vi "configure.vi"(8 "error in (no error)":errorcluster, 11 "DAQmxDigitalOut in":refnum<class "DigitalOutDL110325DAQmx.lvclass">) -> (0 "error out":errorcluster, 3 "DAQmxDigitalOut out":refnum<class "DigitalOutDL110325DAQmx.lvclass">)   [LabVIEW 2010, in "DigitalOutDL110325DAQmx.lvclass"]
doc: "The dynamic dispatch version of this VI loads and displays the configuration file associated with the plug-in object. The user modify and save the configuration data."
uses:
  DigitalOutDL110325DAQmx.lvclass
  DigitalOutDL110325DAQmx.lvclass/DigitalOutDL110325DAQmx.ctl
  common/classes/GenericComponent/GenericComponent/GenericComponent.lvclass
panel:
  out "Configuration":string
  in  "digital output line":tag
  in  "Save Button":bool
  in  "Cancel Button":bool
  # "Configure DAQmxDigitalOut component"
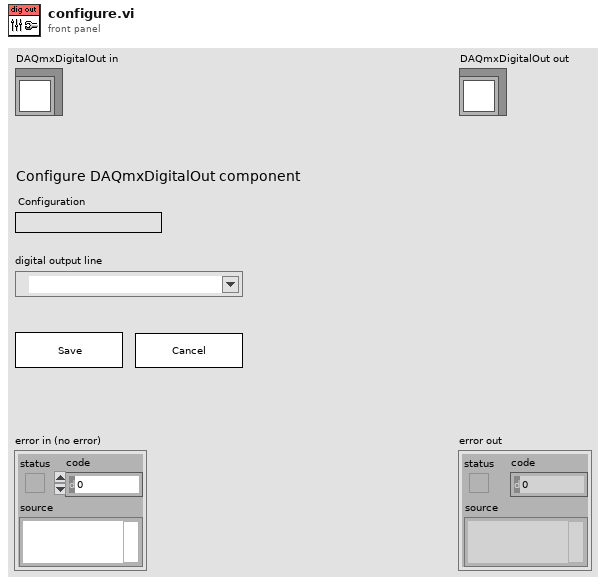
[diagram p1: front panel]
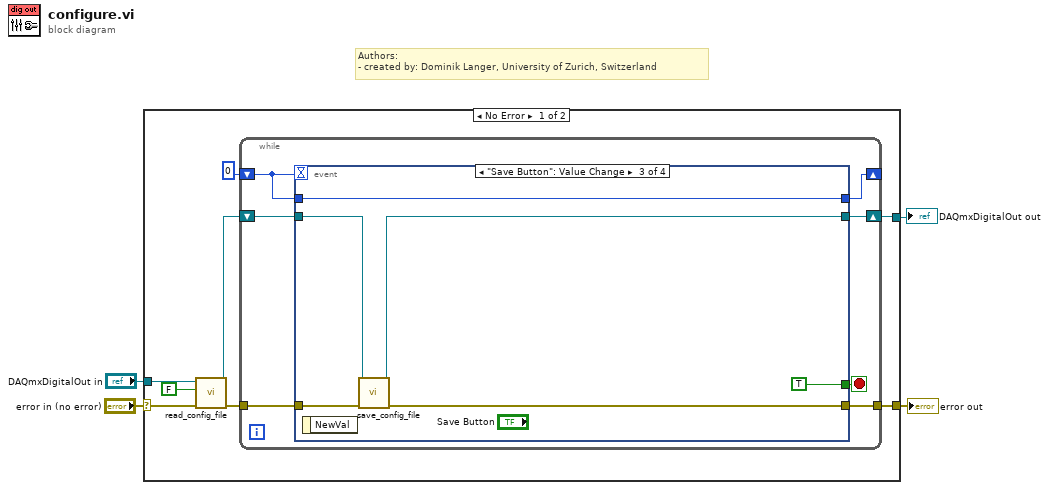
[diagram p0: block diagram]
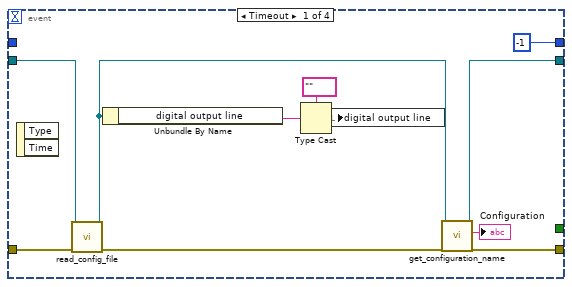
[diagram p2: hidden frame]
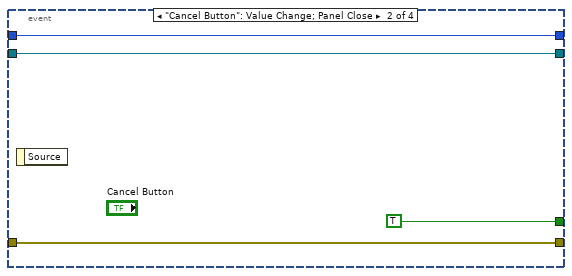
[diagram p3: hidden frame]
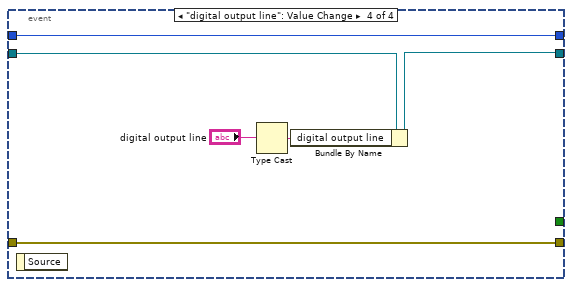
[diagram p4: hidden frame]
diagram:
  # "Authors: \n- created by: Dominik Langer, University of Zurich, Switzerland"
  n1 = case shown="No Error" "error in (no error)" {
    selector: "error in (no error)" -> [w9 w48]
    tunnel: [w12 w48] -> w1
    tunnel: [w10 w47] -> w3
    tunnel: "DAQmxDigitalOut in" -> [w7 w47]
    frame No Error {
      n2 = call-dynamic "read_config_file.vi"("error in (no error)"=w9, "force load?"=FALSE, "GenericPlugin in"=w7) -> ("error out"=w8:errorcluster, "GenericPlugin out"=w6:refnum<class "DigitalOutDL110325DAQmx.lvclass">)  [unwired: 7 out]
      n3 = while {
        tunnel: w8 -> [w19]
        tunnel: [w18] -> w12
        shift-right: [w15] -> _
        shift-left: 0 -> [w16]
        shift-right: [w13] -> w10
        shift-left: w6 -> [w14]
        stop <- w17 stop-if-true
        n4 = event shown="[2] \"Save Button\": Value Change" {
          selector: _ -> [_ _ _ _]
          dyn-events: _ -> [_ _ _ _]
          timeout: w16 -> [_ _ _ _]
          tunnel: w19 -> [w28 w34 w37 w41]
          tunnel: [w23 w34 w38 w41] -> w18
          tunnel: [_ TRUE TRUE _] -> w17
          tunnel: w16 -> [_ w32 w39 w42]
          tunnel: [-1 w32 w39 w42] -> w15
          tunnel: w14 -> [w29 w31 w35 w44]
          tunnel: [w20 w31 w36 w43] -> w13
          event Timeout {
            n5 = event-data() -> ()  [unwired: 3 out]
            n6 = call-dynamic "read_config_file.vi"("error in (no error)"=w28, "GenericPlugin in"=w29) -> ("error out"=w24:errorcluster, "GenericPlugin out"=w21:refnum<class "DigitalOutDL110325DAQmx.lvclass">)  [unwired: 1 in, 7 out]
            n7 = Unbundle By Name(w21) -> ("digital output line"=w27:string)
            n8 = Type Cast(type=tag "" ("shutter digital output line"), x=w27) -> (*(type *) &x=w26:tag)
            n9 = local write "digital output line"(w26) -> ()
            n10 = call "get_configuration_name.vi"("error in (no error)"=w24, "GenericPlugin.lvclass in"=w21) -> ("error out"=w23:errorcluster, "configuration name"=→"Configuration":string, "GenericPlugin.lvclass out"=w20:refnum<class "DigitalOutDL110325DAQmx.lvclass">)  [unwired: 7 in]
          }
          event "Cancel Button": Value Change; Panel Close {
            n11 = event-data() -> ()  [unwired: 2 out]
          }
          event "Save Button": Value Change {
            n12 = event-data() -> ()  [unwired: 2 out]
            n13 = call-dynamic "save_config_file.vi"("error in (no error)"=w37, "GenericPlugin in"=w35) -> ("error out"=w38:errorcluster, "GenericPlugin out"=w36:refnum<class "DigitalOutDL110325DAQmx.lvclass">)  [unwired: 2 in, 6 out]
          }
          event "digital output line": Value Change {
            n14 = event-data() -> ()  [unwired: 2 out]
            n15 = Type Cast(x="digital output line") -> (*(type *) &x=w46:string)  [unwired: 1 out]
            n16 = Bundle By Name(cluster=w44, "digital output line"=w46) -> (w43:refnum<class "DigitalOutDL110325DAQmx.lvclass">)
          }
        }
      }
    }
    frame Error {
    }
  }
  "error out" <- w1
  "DAQmxDigitalOut out" <- w3
